vi "Test View.vi"(10 "User Events in":refnum<class "User Events.lvclass">) -> ()   [LabVIEW 2016, in "FAMT Views.lvlib"]
uses:
  FAMT Views.lvlib
  User Events/User Events.lvclass
  Commands/Command Factory/Command Factory.lvclass
  User Events/User Events.lvclass/User Events.ctl
  Typedefs/StateTypes.ctl
  Commands/Complete Testing Command/Complete Testing Command.lvclass
  Commands/Full Force Test Command/Full Force Test Command.lvclass
  Commands/Operational Force Test Command/Operational Force Test Command.lvclass
  Commands/Differential Pressure Release Valve Test Command/Differential Pressure Release Valve Test Command.lvclass
  Commands/Force Accuracy Test Command/Force Accuracy Test Command.lvclass
  Commands/Sentran Accuracy Test Command/Sentran Accuracy Test Command.lvclass
  Commands/Tracking Test Command/Tracking Test Command.lvclass
  Commands/Slewing Test Command/Slewing Test Command.lvclass
  Typedefs/FAMT Typedefs.lvlib
panel:
  in  "Slewing Test":bool
  in  "Tracking Test":bool
  in  "Sentran Accuracy Test":bool
  in  "Force Accuracy Test":bool
  in  "DPRV Test":bool
  in  "Operational Force Test":bool
  in  "Full Force Test":bool
  in  "CompleteTest":bool
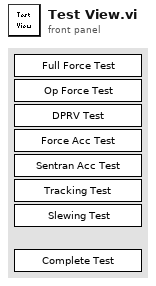
[diagram p1: front panel]
types:
  T1 = typedef "FAMT Typedefs.lvlib/Publish Data Events.ctl" = cluster{"State":refnum<user-event>, "ErrorCode":refnum<user-event>, "Scan Progress":refnum<user-event>}
  T2 = typedef "FAMT Typedefs.lvlib/Subscribe Data Events.ctl" = cluster{"Command":refnum<user-event>}
  T3 = cluster{"Event Registration Refnum":refnum<event-registration>}
  T4 = typedef "FAMT Typedefs.lvlib/StateTypes.ctl" = enum16{"Offline State", "Fault State", "Standby State", "Disabled State", "Enabled State", "Wait For User Input State", "Test Actuator State"}
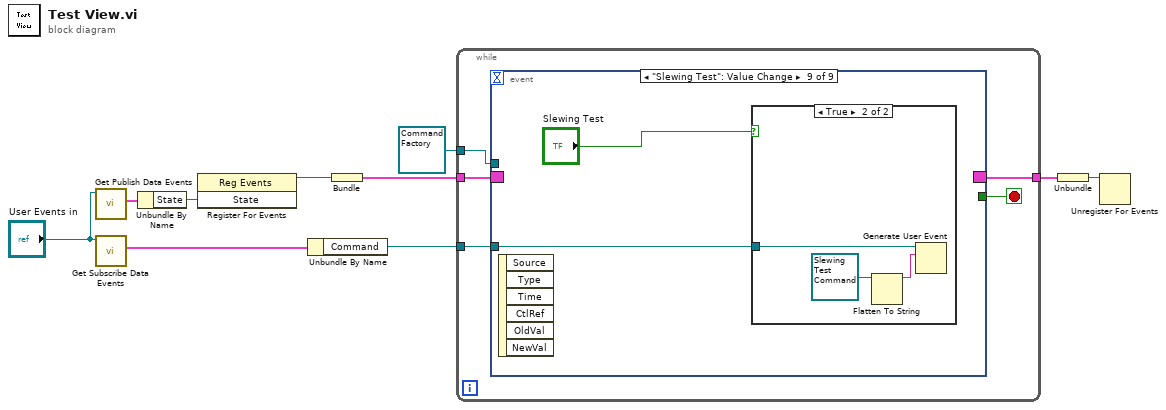
[diagram p0: block diagram]
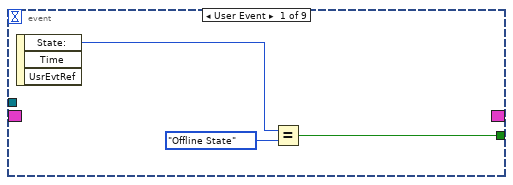
[diagram p2: hidden frame]
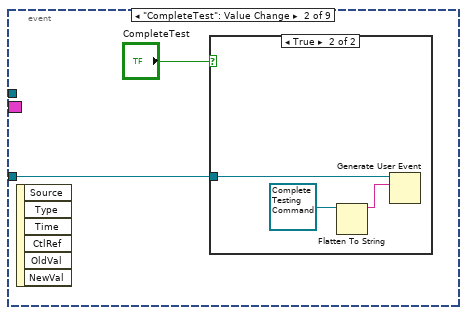
[diagram p3: hidden frame]
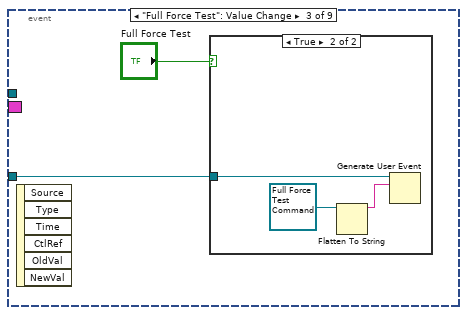
[diagram p5: hidden frame]
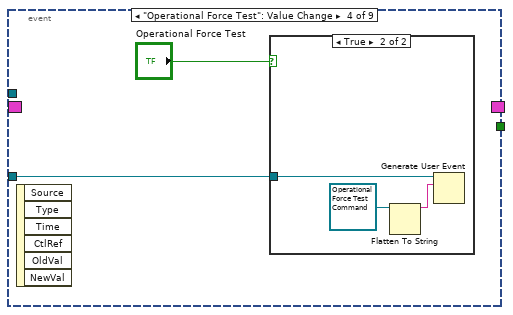
[diagram p7: hidden frame]
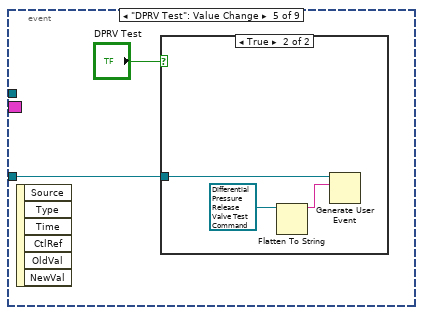
[diagram p9: hidden frame]
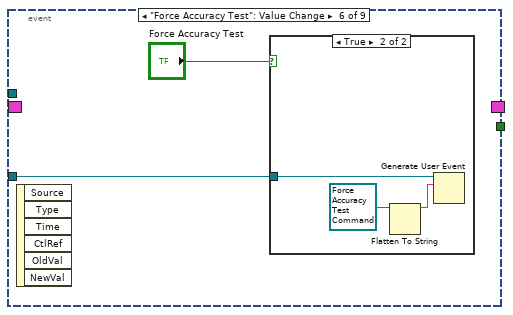
[diagram p11: hidden frame]
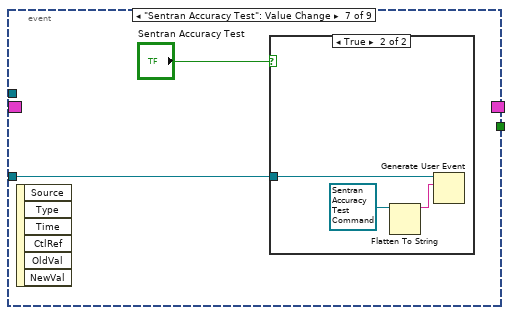
[diagram p13: hidden frame]
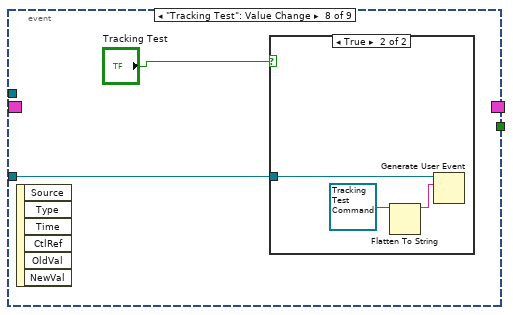
[diagram p15: hidden frame]
diagram:
  n1 = call "Get Publish Data Events.vi"("UserEvents in"="User Events in") -> ("Publish Data Events"=w10:T1)  [unwired: 9 in, 1 out]
  n2 = call "Get Subscribe Data Events.vi"("UserEvents in"="User Events in") -> ("Subscribe Data Events"=w4:T2)  [unwired: 9 in, 1 out]
  n3 = Unbundle By Name(w10) -> ("State"=w9:refnum<user-event>)
  n4 = register-events(w9) -> (reference out=w8:refnum<event-registration>)  [unwired: 2 in, 1 out]
  n5 = Unbundle By Name(w4) -> ("Command"=w2:refnum<user-event>)
  n6 = Bundle("Event Registration Refnum"=w8) -> (w5:T3)  [unwired: 1 in]
  n7 = while {
    tunnel: w5 -> [w15]
    tunnel: [w14] -> w6
    tunnel: w2 -> [w12]
    tunnel: refnum<class "Command Factory.lvclass"> refnum ("CommandFactory.lvclass") -> [w11]
    stop <- w13 stop-if-true
    n8 = event shown="[8] \"Slewing Test\": Value Change" {
      selector: w15 -> [_ _ _ _ _ _ _ _ _]
      dyn-events: [_ _ _ _ _ _ _ _ _] -> w14
      timeout: _ -> [_ _ _ _ _ _ _ _ _]
      tunnel: [w17 _ _ _ _ _ _ _ _] -> w13
      tunnel: w12 -> [_ w19 w25 w30 w35 w40 w45 w50 w55]
      tunnel: w11 -> [_ _ _ _ _ _ _ _ _]
      event User Event {
        n9 = event-data() -> ("State:"=w16:T4)  [unwired: 1 in, 2 out]
        n10 = Equal?(x=w16, y=StateTypes."Offline State") -> (x = y?=w17:bool)
      }
      event "CompleteTest": Value Change {
        n11 = event-data() -> ()  [unwired: 1 in, 6 out]
        n12 = case shown="True" "CompleteTest" {
          tunnel: w19 -> [_ w22]
          frame False {
          }
          frame True {
            n13 = Flatten To String(anything=refnum<class "Complete Testing Command.lvclass"> refnum ("Complete Testing Command.lvclass")) -> (data string=w23:string)  [unwired: 3 in, 2 out]
            n14 = Generate User Event(user event=w22, event data cluster=w23) -> ()  [unwired: 2 in, 2 out]
          }
        }
      }
      event "Full Force Test": Value Change {
        n15 = event-data() -> ()  [unwired: 1 in, 6 out]
        n16 = case shown="True" "Full Force Test" {
          tunnel: w25 -> [_ w27]
          frame False {
          }
          frame True {
            n17 = Flatten To String(anything=refnum<class "Full Force Test Command.lvclass"> refnum ("Full Force Test Command.lvclass")) -> (data string=w28:string)  [unwired: 3 in, 2 out]
            n18 = Generate User Event(user event=w27, event data cluster=w28) -> ()  [unwired: 2 in, 2 out]
          }
        }
      }
      event "Operational Force Test": Value Change {
        n19 = event-data() -> ()  [unwired: 1 in, 6 out]
        n20 = case shown="True" "Operational Force Test" {
          tunnel: w30 -> [_ w32]
          frame False {
          }
          frame True {
            n21 = Flatten To String(anything=refnum<class "Operational Force Test Command.lvclass"> refnum ("Operational Force Test Command.lvclass")) -> (data string=w33:string)  [unwired: 3 in, 2 out]
            n22 = Generate User Event(user event=w32, event data cluster=w33) -> ()  [unwired: 2 in, 2 out]
          }
        }
      }
      event "DPRV Test": Value Change {
        n23 = event-data() -> ()  [unwired: 1 in, 6 out]
        n24 = case shown="True" "DPRV Test" {
          tunnel: w35 -> [_ w37]
          frame False {
          }
          frame True {
            n25 = Flatten To String(anything=refnum<class "Differential Pressure Release Valve Test Command.lvclass"> refnum ("Differential Pressure Release Valve Test Command.lvclass")) -> (data string=w38:string)  [unwired: 3 in, 2 out]
            n26 = Generate User Event(user event=w37, event data cluster=w38) -> ()  [unwired: 2 in, 2 out]
          }
        }
      }
      event "Force Accuracy Test": Value Change {
        n27 = event-data() -> ()  [unwired: 1 in, 6 out]
        n28 = case shown="True" "Force Accuracy Test" {
          tunnel: w40 -> [_ w42]
          frame False {
          }
          frame True {
            n29 = Flatten To String(anything=refnum<class "Force Accuracy Test Command.lvclass"> refnum ("Force Accuracy Test Command.lvclass")) -> (data string=w43:string)  [unwired: 3 in, 2 out]
            n30 = Generate User Event(user event=w42, event data cluster=w43) -> ()  [unwired: 2 in, 2 out]
          }
        }
      }
      event "Sentran Accuracy Test": Value Change {
        n31 = event-data() -> ()  [unwired: 1 in, 6 out]
        n32 = case shown="True" "Sentran Accuracy Test" {
          tunnel: w45 -> [_ w47]
          frame False {
          }
          frame True {
            n33 = Flatten To String(anything=refnum<class "Sentran Accuracy Test Command.lvclass"> refnum ("Sentran Accuracy Test Command.lvclass")) -> (data string=w48:string)  [unwired: 3 in, 2 out]
            n34 = Generate User Event(user event=w47, event data cluster=w48) -> ()  [unwired: 2 in, 2 out]
          }
        }
      }
      event "Tracking Test": Value Change {
        n35 = event-data() -> ()  [unwired: 1 in, 6 out]
        n36 = case shown="True" "Tracking Test" {
          tunnel: w50 -> [_ w52]
          frame False {
          }
          frame True {
            n37 = Flatten To String(anything=refnum<class "Tracking Test Command.lvclass"> refnum ("Tracking Test Command.lvclass")) -> (data string=w53:string)  [unwired: 3 in, 2 out]
            n38 = Generate User Event(user event=w52, event data cluster=w53) -> ()  [unwired: 2 in, 2 out]
          }
        }
      }
      event "Slewing Test": Value Change {
        n39 = event-data() -> ()  [unwired: 1 in, 6 out]
        n40 = case shown="True" "Slewing Test" {
          tunnel: w55 -> [_ w57]
          frame False {
          }
          frame True {
            n41 = Flatten To String(anything=refnum<class "Slewing Test Command.lvclass"> refnum ("Slewing Test Command.lvclass")) -> (data string=w58:string)  [unwired: 3 in, 2 out]
            n42 = Generate User Event(user event=w57, event data cluster=w58) -> ()  [unwired: 2 in, 2 out]
          }
        }
      }
    }
  }
  n43 = Unbundle(w6) -> ("Event Registration Refnum"=w7:refnum<event-registration>)
  n44 = Unregister For Events(event registration refnum=w7) -> ()  [unwired: 1 in, 1 out]
